vi "Write Async Method Error.vi"(8 "error in (no error)":errorcluster, 10 "Async Method Error":errorcluster, 11 "Async Message in":refnum<class "Async Message.lvclass">) -> (0 "error out":errorcluster, 3 "Async Message out":refnum<class "Async Message.lvclass">)   [LabVIEW 2023, in "Async Methods Actor.lvlib" / "Async Message.lvclass"]
uses:
  Async Message.lvclass
  Async Message.lvclass/Async Message.ctl
  Completion Notification Msg/Completion Notification Msg.lvclass/Completion Notification Msg.ctl
  Completion Notification Msg/Completion Notification Msg.lvclass
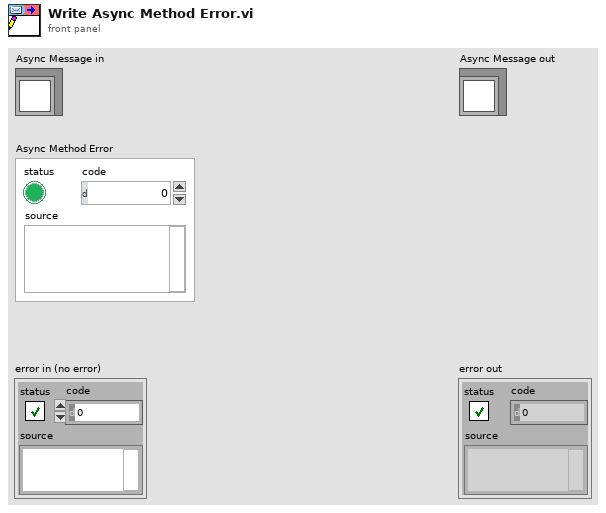
[diagram p1: front panel]
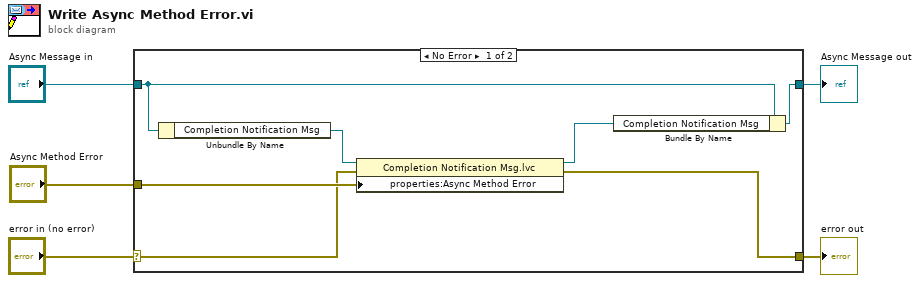
[diagram p0: block diagram]
diagram:
  n1 = case shown="No Error" "error in (no error)" {
    selector: "error in (no error)" -> [w10 w13]
    tunnel: [w9 w13] -> w4
    tunnel: [w8 w14] -> w2
    tunnel: "Async Message in" -> [w7 w14]
    tunnel: "Async Method Error" -> [w11 _]
    frame No Error {
      n2 = Unbundle By Name(w7) -> ("Completion Notification Msg"=w12:refnum<class "Completion Notification Msg.lvclass">)
      n3 = property class="Completion Notification Msg.lvc"(reference=w12, error in=w10, "properties:Async Method Error"=w11) -> (reference out=w6:refnum<class "Completion Notification Msg.lvclass">, error out=w9:errorcluster)
      n4 = Bundle By Name(cluster=w7, "Completion Notification Msg"=w6) -> (w8:refnum<class "Async Message.lvclass">)
    }
    frame Error {
    }
  }
  "error out" <- w4
  "Async Message out" <- w2
